vi "DMM Read.vi"(8 "error in (no error)":errorcluster, 9 "Maximum Time (msec)":i32=-1, 10 "instrument handle":refnum<k15>, 11 "DMM in":refnum<class "DMM.lvclass">) -> (0 "error out":errorcluster, 1 "Measurement":dbl format="%.5f", 2 "instrument handle out":refnum<k15>, 3 "DMM out":refnum<class "DMM.lvclass">)   [LabVIEW 2023, in "HardwareAbstractionLayer_LVOOP.lvlib" / "DMM.lvclass"]
uses:
  DMM.lvclass
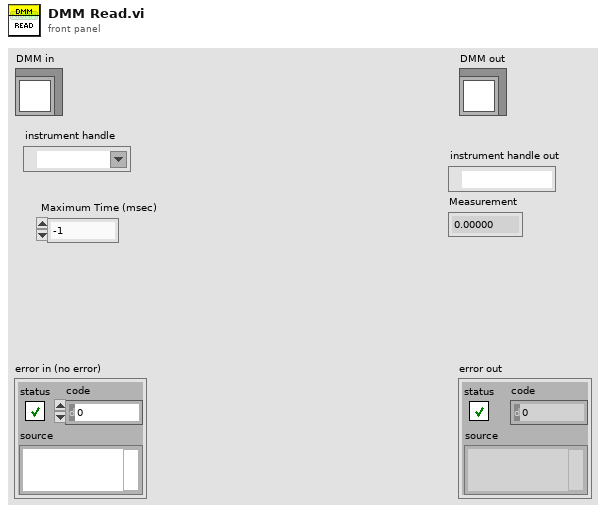
[diagram p1: front panel]
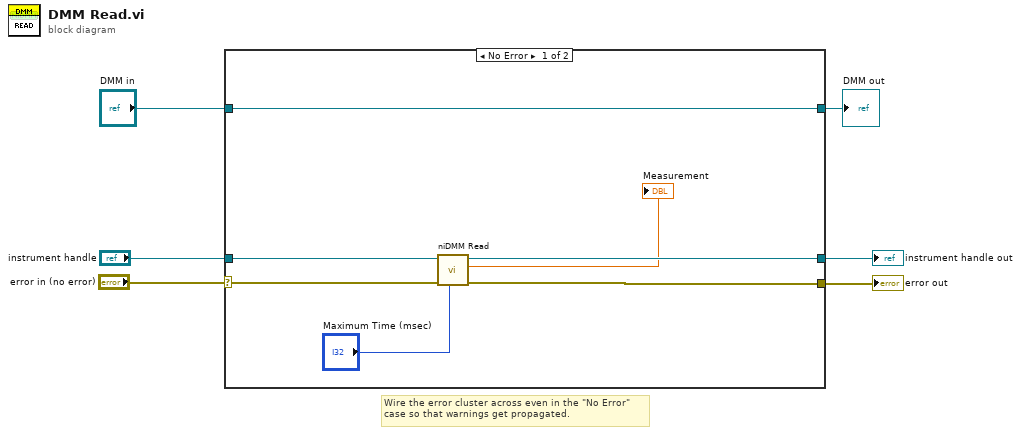
[diagram p0: block diagram]
diagram:
  # "Wire the error cluster across even in the \"No Error\"\ncase so that warnings get propagated."
  n1 = case shown="No Error" "error in (no error)" {
    selector: "error in (no error)" -> [w11 w16]
    tunnel: [w10 w16] -> w5
    tunnel: [w13 w15] -> w3
    tunnel: "DMM in" -> [w13 w15]
    tunnel: "instrument handle" -> [w12 w14]
    tunnel: [w9 w14] -> w1
    frame No Error {
      n2 = call <instrlib>:"niDMM Read.vi"("Maximum Time (msec)"="Maximum Time (msec)", "error in (no error)"=w11, "instrument handle"=w12) -> ("error out"=w10:errorcluster, "Measurement"=→"Measurement":dbl, "instrument handle out"=w9:refnum<k15>)  [unwired: 6 in]
    }
    frame Error {
    }
  }
  "error out" <- w5
  "DMM out" <- w3
  "instrument handle out" <- w1
